vi "ADC exampleKleuren fast.vi"() -> ()   [LabVIEW 2018]
uses:
  FSM States.ctl
panel:
  out "Wit":bool
  out "Rood":bool
  out "Zwart":bool
  in  "digital out":bool[](array[boolean])
  in  "stop 2":bool
  in  "Kleurmaken":bool
  in  "KLEUREN":bool
  out "Beginning State":T1
  out "analog in":dbl[](array[numeric]) format="%0.2f"
  in  "stop":bool
  # "ADC READ EXAMPLE"
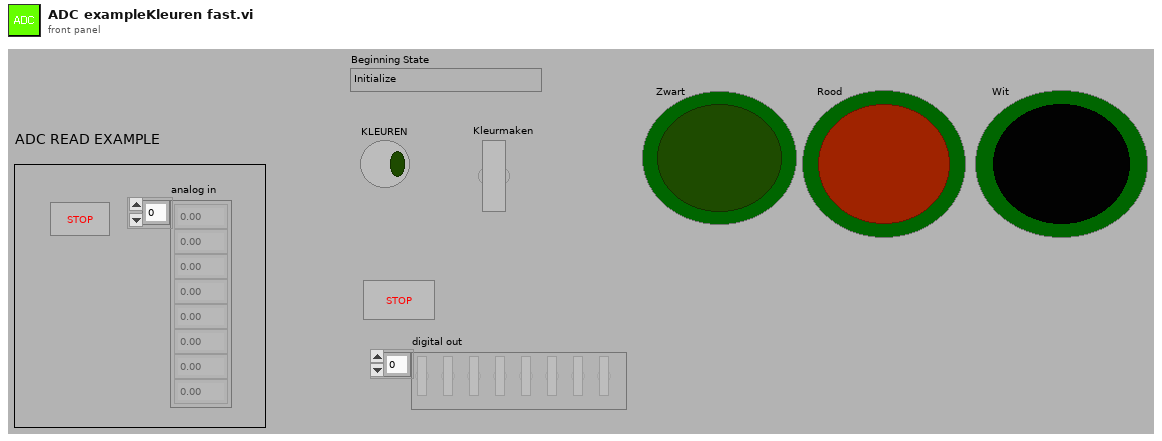
[diagram p1: front panel]
types:
  T1 = typedef "FSM States.ctl" = enum16{"Initialize", "ROOD", "GROEN ", "Blauw "}
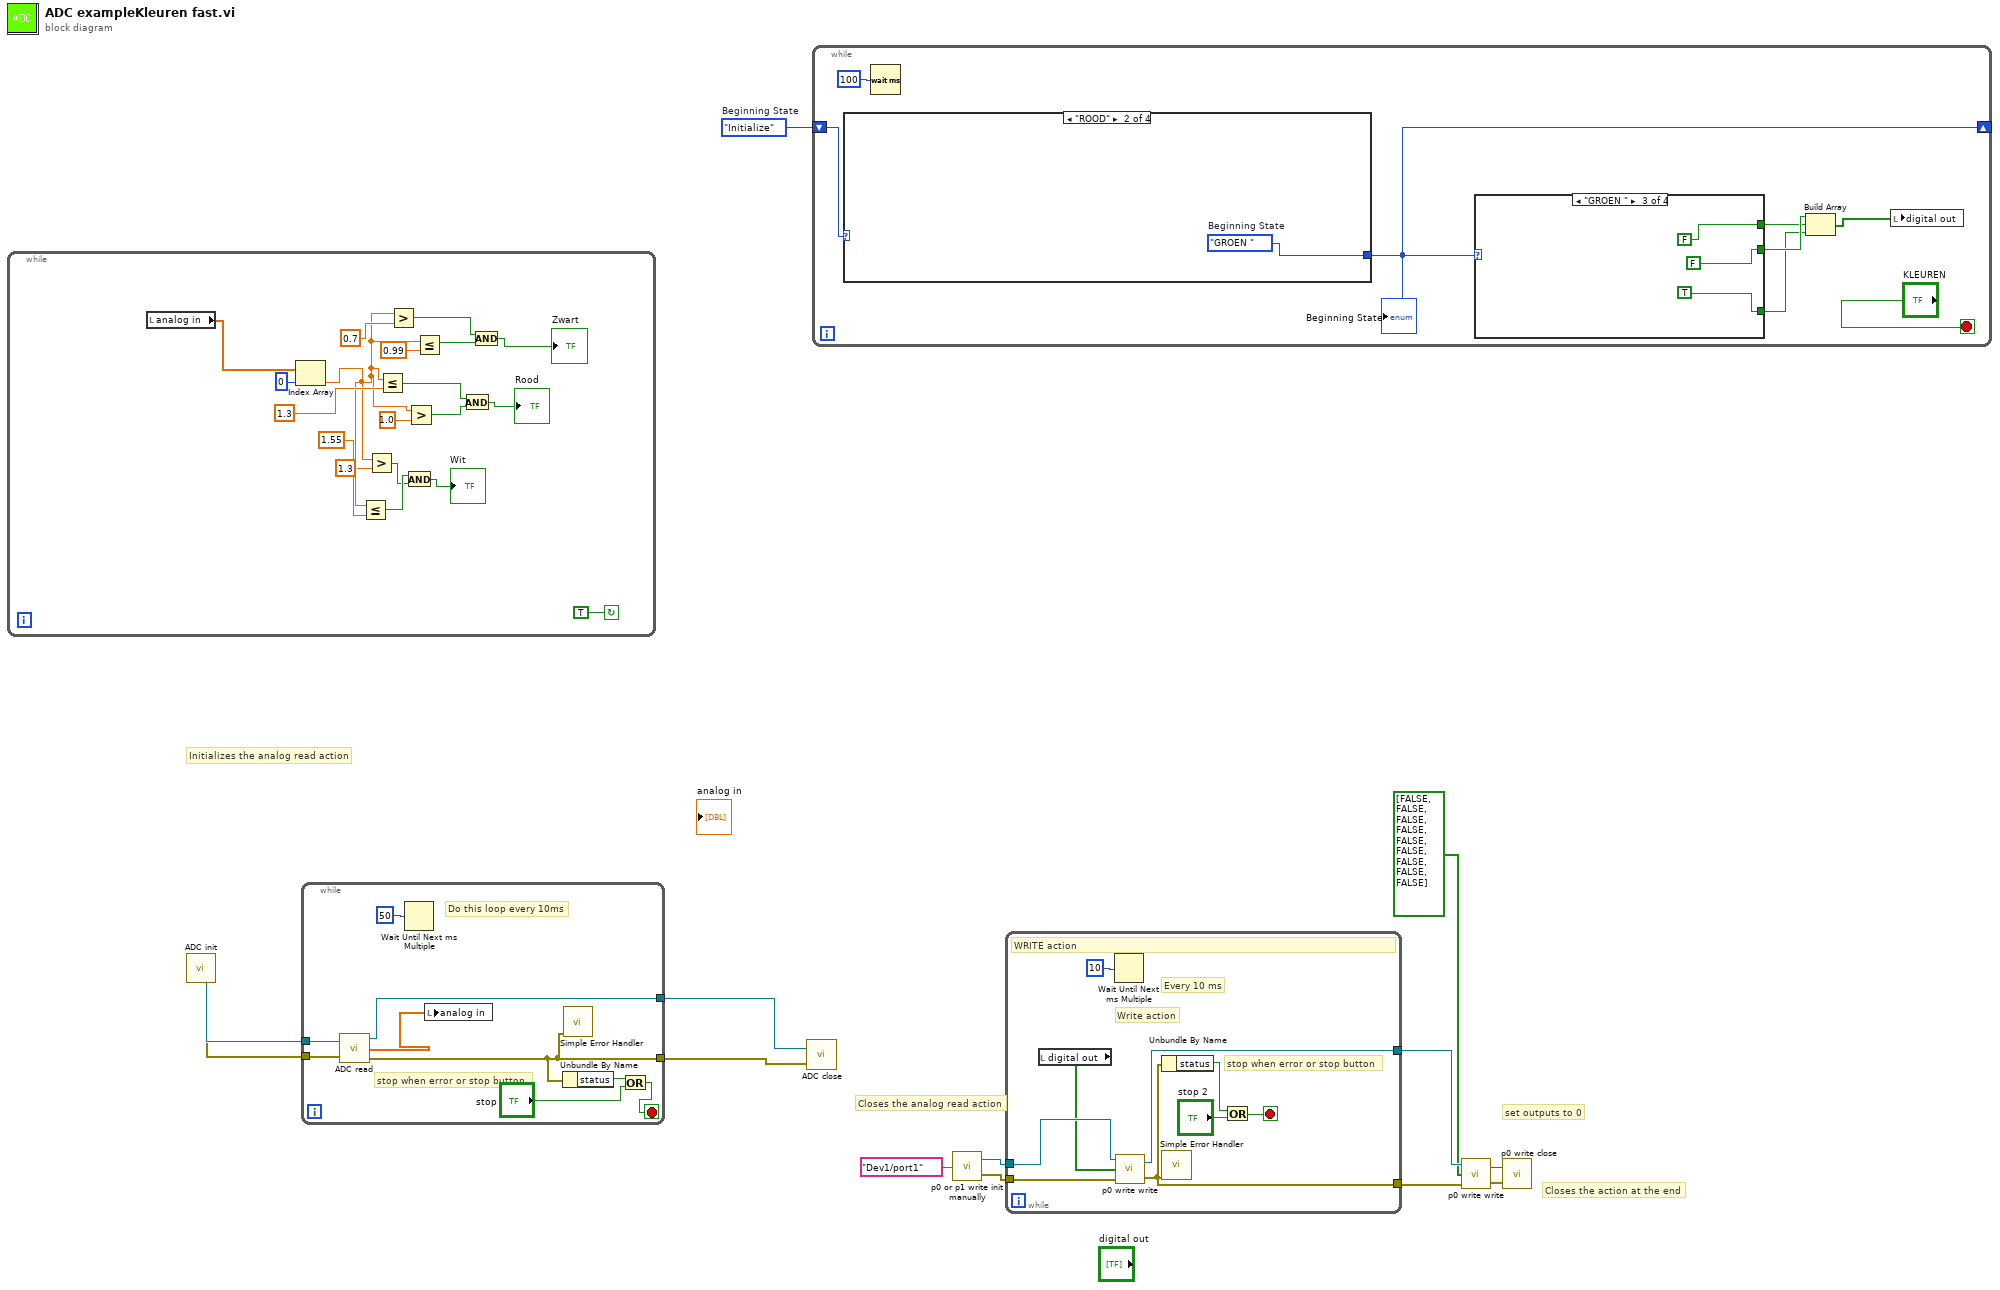
[diagram p0: block diagram]
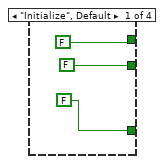
[diagram p2: hidden frame]
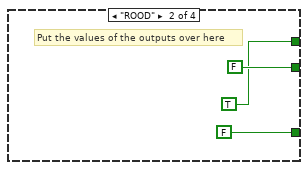
[diagram p3: hidden frame]
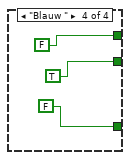
[diagram p4: hidden frame]
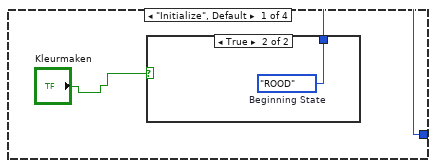
[diagram p5: hidden frame]
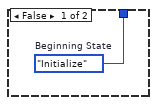
[diagram p6: hidden frame]
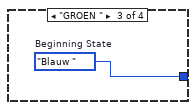
[diagram p7: hidden frame]
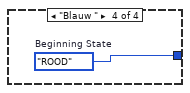
[diagram p8: hidden frame]
diagram:
  w9 = FSM_States."Initialize"  # Beginning State
  # "set outputs to 0"
  # "Closes the action at the end"
  # "Closes the analog read action"
  # "Initializes the analog read action"
  n1 = while {
    stop <- TRUE continue-if-true
    n2 = local read "analog in"() -> (w30:dbl[])
    n3 = Index Array(array=w30, index=0) -> (element=w15:dbl)
    n4 = Less Or Equal?(x=w15, y=1.55) -> (x <= y?=w18:bool)
    n5 = Greater?(x=w15, y=1.3) -> (0:w17:bool)
    n6 = Less Or Equal?(x=w15, y=1.3) -> (x <= y?=w20:bool)
    n7 = Greater?(x=w15, y=0.7) -> (0:w26:bool)
    n8 = And(x=w18, y=w17) -> (x .and. y?=→"Wit":bool)
    n9 = Greater?(x=w15, y=1.0) -> (0:w19:bool)
    n10 = Less Or Equal?(x=w15, y=0.99) -> (x <= y?=w25:bool)
    n11 = And(x=w20, y=w19) -> (x .and. y?=→"Rood":bool)
    n12 = And(x=w26, y=w25) -> (x .and. y?=→"Zwart":bool)
  }
  n13 = call "ADC init.vi"() -> ("error out"=w12:errorcluster, "task out"=w13:refnum<k21>)
  n14 = while {
    tunnel: w13 -> [w41]
    tunnel: w12 -> [w40]
    tunnel: [w37] -> w11
    tunnel: [w39] -> w10
    stop <- w34 stop-if-true
    # "stop when error or stop button"
    # "Do this loop every 10ms"
    n15 = call "ADC read.vi"("task/channels in"=w41, "error in"=w40) -> ("task out"=w39:refnum<k21>, "analog in"=w33:dbl[], "error out"=w37:errorcluster)
    n16 = Wait Until Next ms Multiple(millisecond multiple=u32 50) -> ()  [unwired: 1 out]
    n17 = local write "analog in"(w33) -> ()
    n18 = Unbundle By Name(w37) -> ("status"=w36:bool)
    n19 = call <vilib>:"Simple Error Handler.vi"("error in (no error)"=w37) -> ()  [unwired: 4 in, 5 out]
    n20 = Or(x=w36, y="stop") -> (x .or. y?=w34:bool)
  }
  n21 = call "ADC close.vi"("error in"=w11, "task/channels in"=w10) -> ()
  n22 = while {
    shift-right: [w42] -> _
    shift-left: w9 -> [w49]
    stop <- "KLEUREN" stop-if-true
    n23 = case shown="\"ROOD\"" w49 {
      tunnel: [w63 w66 w67 w68] -> w42
      frame "Initialize", Default {
        n24 = case shown="True" "Kleurmaken" {
          tunnel: [w64 w65] -> w63
          frame False {
            w64 = FSM_States."Initialize"  # Beginning State
          }
          frame True {
            w65 = FSM_States."ROOD"  # Beginning State
          }
        }
      }
      frame "ROOD" {
        w66 = FSM_States."GROEN "  # Beginning State
      }
      frame "GROEN " {
        w67 = FSM_States."Blauw "  # Beginning State
      }
      frame "Blauw " {
        w68 = FSM_States."ROOD"  # Beginning State
      }
    }
    "Beginning State" <- w42
    n25 = Wait (ms)(milliseconds to wait=u32 100) -> ()  [unwired: 1 out]
    n26 = case shown="\"GROEN \"" w42 {
      tunnel: [FALSE FALSE FALSE TRUE] -> w45
      tunnel: [FALSE TRUE FALSE FALSE] -> w44
      tunnel: [FALSE FALSE TRUE FALSE] -> w43
      frame "Initialize", Default {
      }
      frame "ROOD" {
        # "Put the values of the outputs over here"
      }
      frame "GROEN " {
      }
      frame "Blauw " {
      }
    }
    n27 = Build Array(w45, w44, w43) -> (w46:bool[])
    n28 = local write "digital out"(w46) -> ()
  }
  n29 = call "p0 or p1 write init manually.vi"("Port"=tag "Dev1/port1") -> ("task out"=w3:refnum<k21>, "error out"=w2:errorcluster)
  n30 = while {
    tunnel: w3 -> [w77]
    tunnel: [w76] -> w8
    tunnel: w2 -> [w75]
    tunnel: [w71] -> w7
    stop <- w72 stop-if-true
    # "stop when error or stop button"
    # "Every 10 ms"
    # "Write action"
    # "WRITE action"
    n31 = local read "digital out"() -> (w69:bool[])
    n32 = Wait Until Next ms Multiple(millisecond multiple=u32 10) -> ()  [unwired: 1 out]
    n33 = call "p0 write write.vi"("error in"=w75, "digital out"=w69, "task/channels in"=w77) -> ("error out"=w71:errorcluster, "task out"=w76:refnum<k21>)
    n34 = Unbundle By Name(w71) -> ("status"=w70:bool)
    n35 = call <vilib>:"Simple Error Handler.vi"("error in (no error)"=w71) -> ()  [unwired: 4 in, 5 out]
    n36 = Or(x=w70, y="stop 2") -> (x .or. y?=w72:bool)
  }
  n37 = call "p0 write write.vi"("error in"=w7, "digital out"=bool[] [FALSE, FALSE, FALSE, FALSE, FALSE, FALSE, FALSE, FALSE, FALSE], "task/channels in"=w8) -> ("error out"=w5:errorcluster, "task out"=w6:refnum<k21>)
  n38 = call "p0 write close.vi"("error in"=w5, "task/channels in"=w6) -> ()
